vi "DSF.Engine.Memory.Cache.Framework.Get Largest Count.All Types.vi"(8 "error in (no error)":errorcluster, 11 "Framework Cache in":refnum<class "DSF.Engine.Memory.Cache.Framework.lvclass">) -> (0 "error out":errorcluster, 2 "Data Type Counts out":T1 {"U64" format="%d elements"; "U32" format="%d elements"; "U16" format="%d elements"; "U8" format="%d elements"; "I64" format="%d elements"; "I32" format="%d elements"; "I16" format="%d elements"; "I8" format="%d elements"; "DBL" format="%d elements"; "SGL" format="%d elements"; "Bool" format="%d elements"}, 3 "Framework Cache out":refnum<class "DSF.Engine.Memory.Cache.Framework.lvclass">)   [LabVIEW 2016, in "DSF.Engine.lvlib" / "DSF.Engine.Memory.Cache.Framework.lvclass"]
uses:
  Cache/DSF.Engine.Memory.Cache.Framework.lvclass
  Typedefs/DSF.Shared.Data Type Counts.ctl
  Cache/DSF.Engine.Memory.Cache.Framework.lvclass/DSF.Engine.Memory.Cache.Framework.ctl
  DSF.Engine.Memory.Cache.Plugin.lvclass/DSF.Engine.Memory.Cache.Plugin.ctl
  DSF.Engine.Memory.Cache.Transfer.lvclass/DSF.Engine.Memory.Cache.Transfer.ctl
  DSF.Engine.Memory.Cache.Plugin.Get Transfer Caches.vi
  DSF.Engine.Memory.Cache.Transfer.Get Largest Count.All Types.vi
  DSF.Engine.Memory.Cache.Transfer.Get Channel Configuration.vi
  DSF.Engine.Memory.Cache.Plugin.lvclass
  DSF.Shared.lvlib
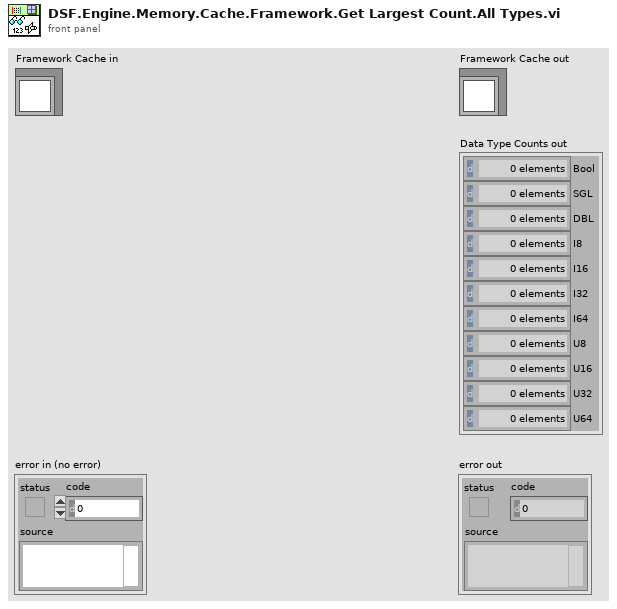
[diagram p1: front panel]
types:
  T1 = typedef "DSF.Shared.lvlib/DSF.Shared.Data Type Counts.ctl" = cluster{"Bool":u64, "SGL":u64, "DBL":u64, "I8":u64, "I16":u64, "I32":u64, "I64":u64, "U8":u64, "U16":u64, "U32":u64, "U64":u64}
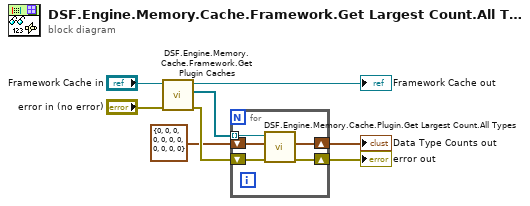
[diagram p0: block diagram]
diagram:
  n1 = call "DSF.Engine.Memory.Cache.Framework.Get Plugin Caches.vi"("error in (no error)"="error in (no error)", "Framework Cache in"="Framework Cache in") -> ("error out"=w4:errorcluster, "Plugin Caches"=w5:refnum<class "DSF.Engine.Memory.Cache.Plugin.lvclass">[], "Framework Cache out"=→"Framework Cache out":refnum<class "DSF.Engine.Memory.Cache.Framework.lvclass">)  [unwired: 7 in]
  n2 = for {
    shift-right: [w13] -> w1
    shift-left: T1 {"Bool"=0, "SGL"=0, "DBL"=0, "I8"=0, "I16"=0, "I32"=0, "I64"=0, "U8"=0, "U16"=0, "U32"=0, "U64"=0} ("Data Type Counts in") -> [w10]
    tunnel: w5 -> [w9] mode=indexing
    shift-right: [w12] -> w3
    shift-left: w4 -> [w11]
    n3 = call "DSF.Engine.Memory.Cache.Plugin.Get Largest Count.All Types.vi"("error in (no error)"=w11, "Data Type Counts in"=w10, "Plugin Cache in"=w9) -> ("error out"=w12:errorcluster, "Data Type Counts out"=w13:T1)  [unwired: 6 in, 1 out]
  }
  "error out" <- w3
  "Data Type Counts out" <- w1
